vi "设备配置界面.vi"() -> ()   [LabVIEW 2016, in "环境动力监测库.lvlib"]
panel:
  in  "配置说明":bool
  in  "设置默认配置":bool
  in  "一键恢复默认设置":bool
  in  "add2":bool
  in  "串口连接":T1(ring)
  in  "设备列表":i32(listbox)=-1
  in  "add":bool
  in  "IO连接":T2(ring)
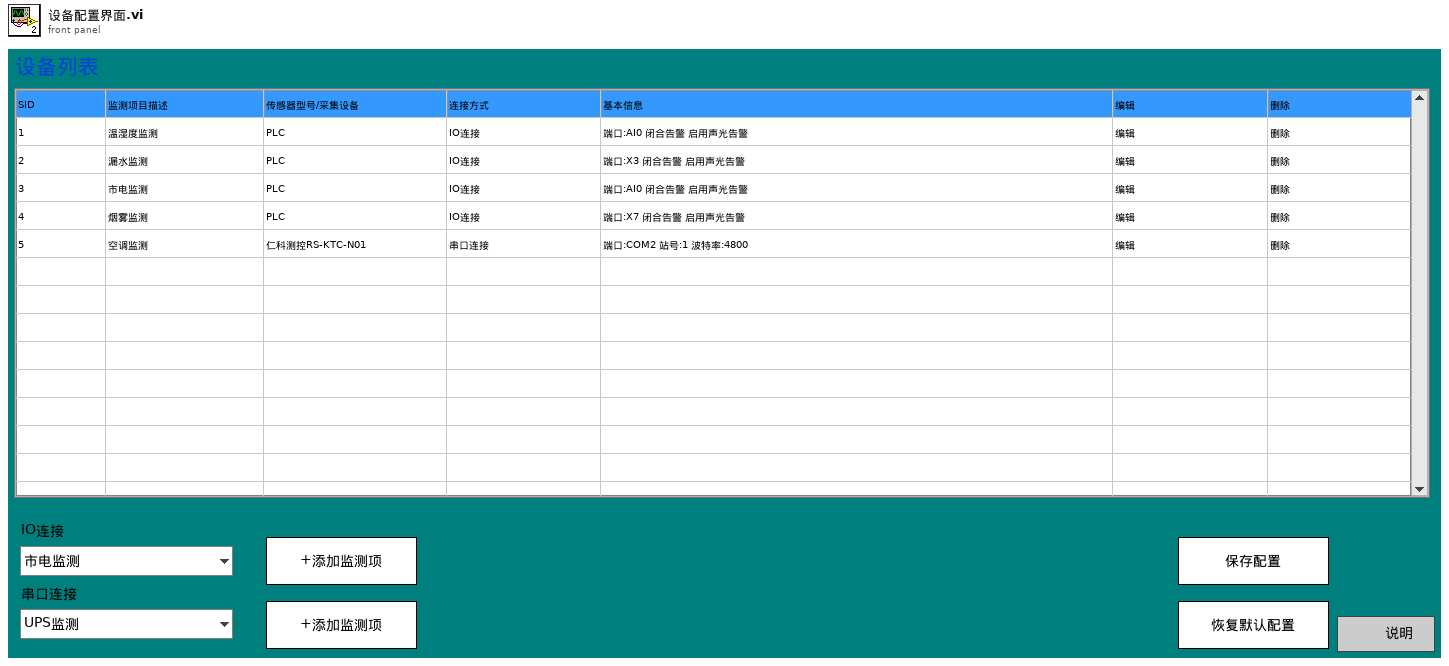
[diagram p1: front panel]
types:
  T1 = enum16{"UPS监测", "空调监测", "蓄电池监测", "GPS监测", "北斗监测", "智能门禁监测"}
  T2 = enum16{"市电监测", "用水量监测", "烟雾监测", "温湿度监测", "振动监测", "红外入侵监测", "漏水监测", "门禁开关监测", "视频监测", "冰箱监测", "排气扇监测"}
  T3 = cluster{"监测项描述:输出":string, "端口":enum16{"AI0", "AI1", "AI2", "AI3", "AI4", "DI0", "DI1", "DI2", "DI3", "DI4", "DO0", "DO1", "DO2", "DO3", "DO4", "X0", "X1", "X2", "X3", "X4", "X5", "X6", "X7", "X8", "X9", "X10", "X11", "X12", "X13", "X14", "X15", "X16", "X17", "X18", "X19", "X20", "X21", "X22", "X23"}, "告警方式":enum32{"禁用告警", "闭合告警", "断开告警"}, "传感器型号":enum16{"PLC", "ZLAN", "ART"}, "声光告警启用":bool}
  T4 = enum16{"AI0", "AI1", "AI2", "AI3", "AI4", "DI0", "DI1", "DI2", "DI3", "DI4", "DO0", "DO1", "DO2", "DO3", "DO4", "X0", "X1", "X2", "X3", "X4", "X5", "X6", "X7", "X8", "X9", "X10", "X11", "X12", "X13", "X14", "X15", "X16", "X17", "X18", "X19", "X20", "X21", "X22", "X23"}
  T5 = cluster{"监测项描述:输出":string, "连接方式":enum16{"串口", "TCP"}, "端口":string, "IP address:":string, "Port:":string, "站号":u64, "传感器型号":string, "波特率":u64, "data bits":u64, "停止位":u16, "奇偶校验":u16, "声光告警启用":bool}
  T6 = typedef "LVPoint32TypeDef.ctl" = cluster{"Horizontal":i32, "Vertical":i32}
  T7 = typedef "LVRowAndColumnTypeDef.ctl" = cluster{"Row":i32, "Column":i32}
  T8 = enum16{"Left Button", "Center Button", "Right Button", "Window Close"}
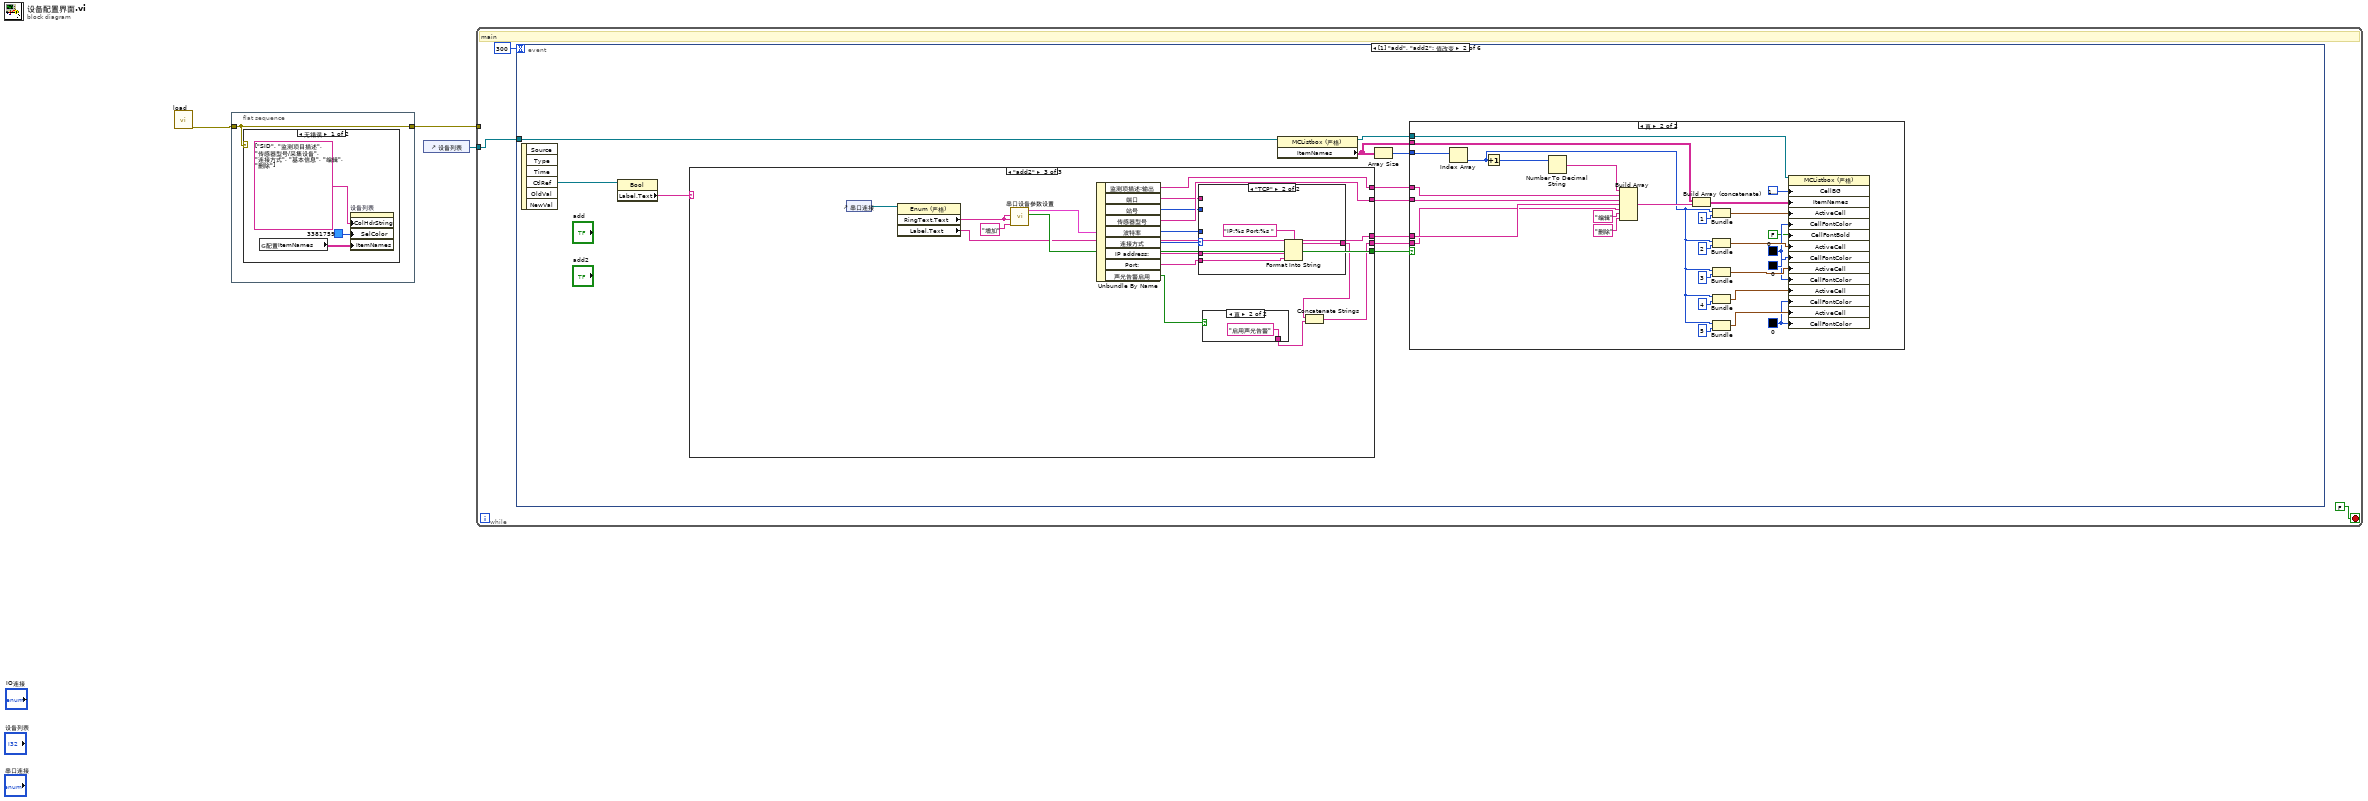
[diagram p0: block diagram]
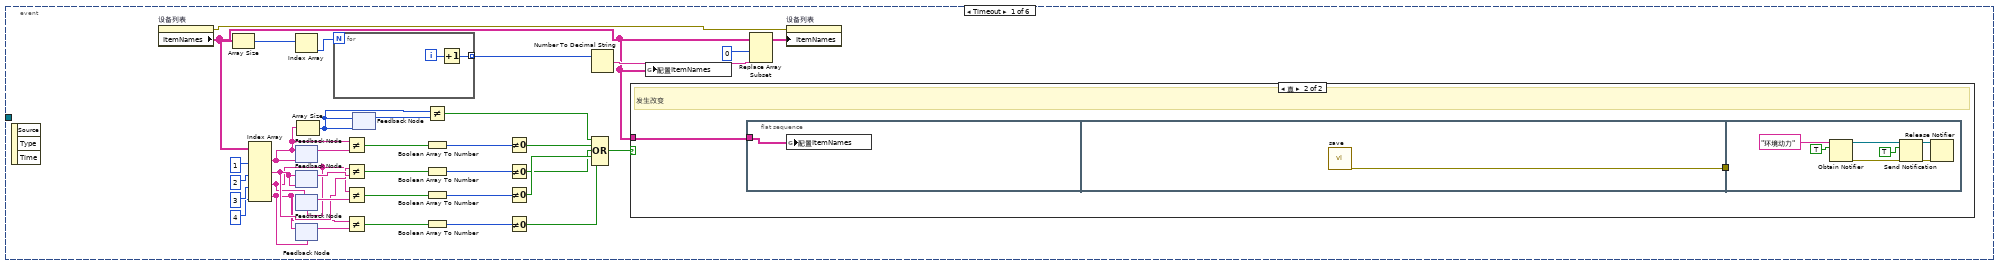
[diagram p3: hidden frame]
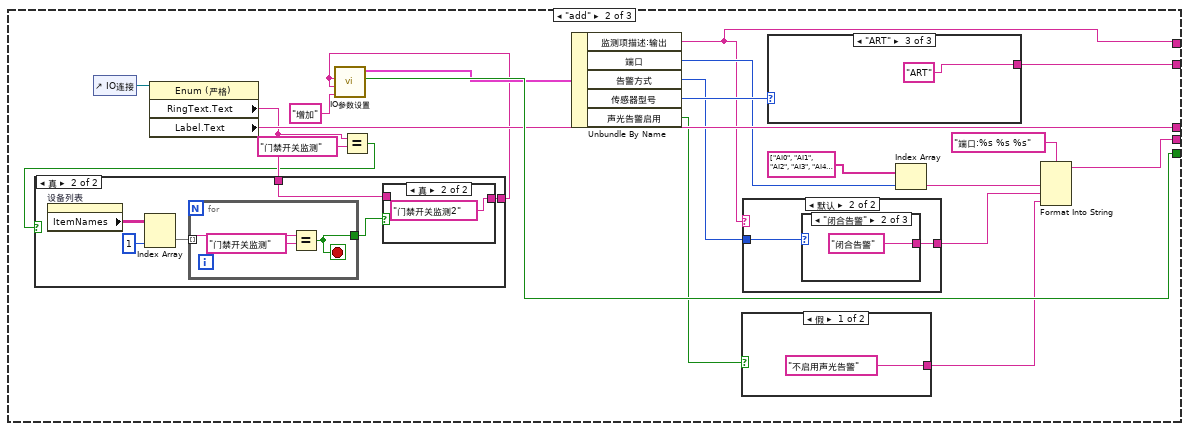
[diagram p6: hidden frame]
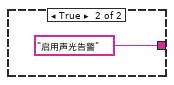
[diagram p7: hidden frame]
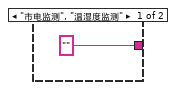
[diagram p10: hidden frame]
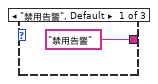
[diagram p11: hidden frame]
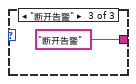
[diagram p12: hidden frame]
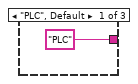
[diagram p13: hidden frame]
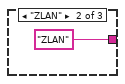
[diagram p14: hidden frame]
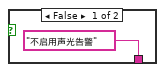
[diagram p15: hidden frame]
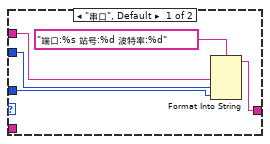
[diagram p16: hidden frame]
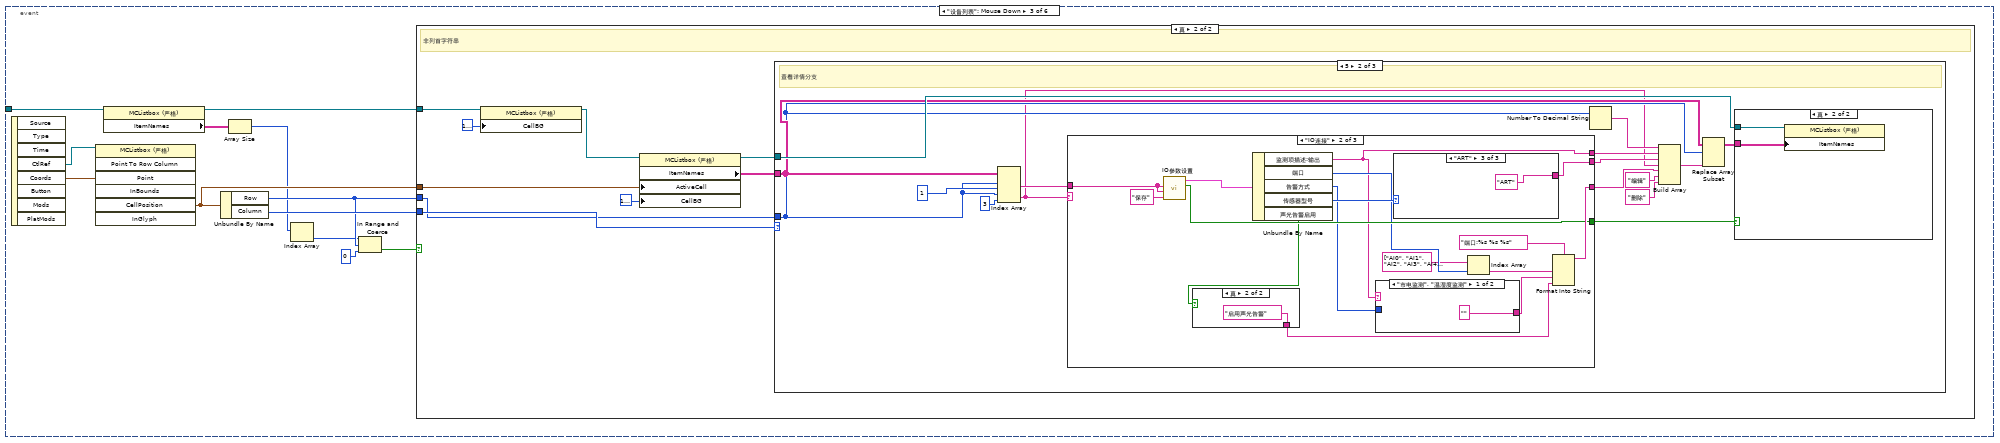
[diagram p18: hidden frame]
diagram:
  n1 = call "load.vi"() -> ("error out"=w1:errorcluster)  [unwired: 11 in]
  n2 = flat-sequence {
    tunnel: w1 -> [w4]
    tunnel: [w4] -> w2
    frame #0 {
      n3 = case shown="无错误" w4 {
        frame No Error {
          n4 = global read "断电保存全局变量.vi" "配置ItemNames"() -> (w5:string[][])
          n5 = property on="设备列表" class="MCListbox (严格)"("ColHdrString"=string[] ["SID", "监测项目描述", "传感器型号/采集设备", "连接方式", "基本信息", "编辑", "删除"] ("列首字符串[]"), "SelColor"=u32 3381759, "ItemNames"=w5) -> ()  [unwired: 2 in, 2 out]
        }
        frame Error {
        }
      }
    }
  }
  n6 = control-ref of="设备列表"() -> (w3:refnum<vi>)
  n7 = while {
    tunnel: w3 -> [w9]
    tunnel: w2 -> [_]
    stop <- FALSE stop-if-true
    # "main"
    n8 = event shown="[1] \"add\", \"add2\": 值改变" {
      selector: _ -> [_ _ _ _ _ _]
      dyn-events: _ -> [_ _ _ _ _ _]
      timeout: 300 -> [_ _ _ _ _ _]
      tunnel: w9 -> [_ w70 w178 _ _ _]
      event Timeout {
        n9 = event-data() -> ()  [unwired: 1 in, 3 out]
        n10 = property on="设备列表" class="MCListbox (严格)"() -> (error out=w45:errorcluster, "ItemNames"=w11:string[][])  [unwired: 2 in, 1 out]
        n11 = Array Size(array=w11) -> (size(s)=w46:i32[])
        n12 = Index Array(array=w11, index (col) #1=1 ("禁用的索引 (列)"), index (col) #2=2 ("索引 (列)"), index (col) #3=3 ("索引 (列)"), index (col) #4=4 ("索引 (列)")) -> (element #1=w16:string[], element #2=w23:string[], element #3=w22:string[], element #4=w21:string[])  [unwired: 4 in]
        n13 = Index Array(array=w46) -> (element=w40:i32)  [unwired: 1 in]
        n14 = feedback-in #1(w16) -> ()
        n15 = feedback #1(w16) -> (w35:string[])
        n16 = feedback #2(w23) -> (w30:string[])
        n17 = feedback-in #2(w23) -> ()
        n18 = feedback #3(w22) -> (w29:string[])
        n19 = feedback-in #3(w22) -> ()
        n20 = feedback #4(w21) -> (w24:string[])
        n21 = feedback-in #4(w21) -> ()
        n22 = Array Size(array=w16) -> (size(s)=w14:i32)
        n23 = for {
          N: w40 -> [_]
          tunnel: [w58] -> w44 mode=indexing
          i -> [w59]
          n24 = Increment(x=w59) -> (x+1=w58:i32)
        }
        n25 = Not Equal?(x=w16, y=w35) -> (x != y?=w15:bool[])
        n26 = Not Equal?(x=w23, y=w30) -> (x != y?=w31:bool[])
        n27 = Not Equal?(x=w22, y=w29) -> (x != y?=w28:bool[])
        n28 = Not Equal?(x=w21, y=w24) -> (x != y?=w25:bool[])
        n29 = feedback #5(w14) -> (w13:i32)
        n30 = feedback-in #5(w14) -> ()
        n31 = Not Equal?(x=w14, y=w13) -> (x != y?=w12:bool)
        n32 = Boolean Array To Number(Boolean array=w15) -> (number=w34:u32)
        n33 = Boolean Array To Number(Boolean array=w31) -> (number=w32:u32)
        n34 = Boolean Array To Number(Boolean array=w28) -> (number=w27:u32)
        n35 = Boolean Array To Number(Boolean array=w25) -> (number=w26:u32)
        n36 = Not Equal To 0?(x=w34) -> (x != 0?=w33:bool)
        n37 = Not Equal To 0?(x=w32) -> (x != 0?=w18:bool)
        n38 = Not Equal To 0?(x=w27) -> (x != 0?=w19:bool)
        n39 = Not Equal To 0?(x=w26) -> (x != 0?=w20:bool)
        n40 = Number To Decimal String(number=w44) -> (decimal integer string=w43:string[])  [unwired: 1 in]
        n41 = Compound Arithmetic op=OR ("复合运算")(w12, w33, w18, w19, w20) -> (w17:bool)
        n42 = case shown="真" w17 {
          tunnel: w11 -> [_ w48]
          frame False {
          }
          frame True {
            # "发生改变"
            n43 = flat-sequence {
              tunnel: w48 -> [w49]
              tunnel: [w50] -> w47
              tunnel: w47 -> [_]
              frame #0 {
                n44 = global write "断电保存全局变量.vi" "配置ItemNames"(w49) -> ()
              }
              frame #1 {
                n45 = call "save.vi"() -> ("error out"=w50:errorcluster)  [unwired: 11 in]
              }
              frame #2 {
                n46 = Obtain Notifier(name (unnamed)="环境动力" ("名称（未命名）"), notification data type=TRUE) -> (notifier out=w53:refnum<notifier>, error out=w54:errorcluster)  [unwired: 2 in, 1 out]
                n47 = Send Notification(notification=TRUE ("通知"), notifier=w53, error in (no error)=w54) -> (notifier out=w56:refnum<notifier>, error out=w57:errorcluster)
                n48 = Release Notifier(notifier=w56, error in (no error)=w57) -> ()  [unwired: 1 in, 3 out]
              }
            }
          }
        }
        n49 = global write "断电保存全局变量.vi" "配置ItemNames"(w11) -> ()
        n50 = Replace Array Subset(array=w11, new element=w43, index (col)=0 ("禁用的索引 (列)")) -> (w41:string[][])  [unwired: 1 in]
        n51 = property on="设备列表" class="MCListbox (严格)"(error in=w45, "ItemNames"=w41) -> ()  [unwired: 1 in, 2 out]
      }
      event "add", "add2": Value Change {
        n52 = event-data() -> ("CtlRef"=w65:refnum<vi>)  [unwired: 1 in, 5 out]
        n53 = property class="Bool"(reference=w65) -> ("Label.Text"=w64:string)  [unwired: 1 in, 2 out]
        n54 = case shown="\"add2\"" w64 {
          tunnel: [_ w91 w131] -> w67
          tunnel: [_ w88 w128] -> w63
          tunnel: [_ w78 w126] -> w62
          tunnel: [_ w83 w125] -> w61
          tunnel: [_ w85 w115] -> w60
          frame "假", Default {
          }
          frame "add" {
            n55 = control-ref of="IO连接"() -> (w89:refnum<vi>)
            n56 = property class="Enum (严格)"(reference=w89) -> ("RingText.Text"=w75:string, "Label.Text"=w88:string)  [unwired: 1 in, 2 out]
            n57 = Equal?(x=w75, y="门禁开关监测") -> (x = y?=w74:bool)
            n58 = case shown="真" w74 {
              tunnel: [w94 w97] -> w77
              tunnel: w75 -> [w94 w96]
              frame False {
              }
              frame True {
                n59 = property on="设备列表" class="MCListbox (严格)"() -> ("ItemNames"=w100:string[][])  [unwired: 2 in, 2 out]
                n60 = Index Array(array=w100, index (col)=1 ("禁用的索引 (列)")) -> (element=w98:string[])  [unwired: 1 in]
                n61 = for {
                  tunnel: w98 -> [w105] mode=indexing
                  tunnel: [w103] -> w95
                  stop <- w103 stop-if-true
                  n62 = Equal?(x=w105, y="门禁开关监测") -> (x = y?=w103:bool)
                }
                n63 = case shown="真" w95 {
                  tunnel: w96 -> [w101 _]
                  tunnel: [w101 "门禁开关监测2" ("y")] -> w97
                  frame False {
                  }
                  frame True {
                  }
                }
              }
            }
            n64 = call "IO参数设置.vi"("布尔文本.文本"="增加", "section (optional)"=w77, "监测项描述"=w77) -> ("增加？"=w91:bool, "簇1输出"=w87:T3)  [unwired: 7 in]
            n65 = Unbundle By Name(w87) -> ("监测项描述:输出"=w78:string, "端口"=w82:T4, "告警方式"=w80:enum32{"禁用告警", "闭合告警", "断开告警"}, "传感器型号"=w84:enum16{"PLC", "ZLAN", "ART"}, "声光告警启用"=w73:bool)
            n66 = case shown="假" w73 {
              tunnel: ["不启用声光告警" "启用声光告警"] -> w72
              frame False {
              }
              frame True {
              }
            }
            n67 = case shown="默认" w78 {
              tunnel: w80 -> [_ w108]
              tunnel: ["" w107] -> w79
              frame "市电监测", "温湿度监测" {
              }
              frame Default {
                n68 = case shown="\"闭合告警\"" w108 {
                  tunnel: ["禁用告警" "闭合告警" "断开告警"] -> w107
                  frame "禁用告警", Default {
                  }
                  frame "闭合告警" {
                  }
                  frame "断开告警" {
                  }
                }
              }
            }
            n69 = case shown="\"ART\"" w84 {
              tunnel: ["PLC" "ZLAN" "ART"] -> w83
              frame "PLC", Default {
              }
              frame "ZLAN" {
              }
              frame "ART" {
              }
            }
            n70 = Index Array(array=string[] ["AI0", "AI1", "AI2", "AI3", "AI4", "DI0", "DI1", "DI2", "DI3", "DI4", "DO0", "DO1", "DO2", "DO3", "DO4", "X0", "X1", "X2", "X3", "X4", "X5", "X6", "X7", "X8", "X9", "X10", "X11", "X12", "X13", "X14", "X15", "X16", "X17", "X18", "X19", "X20", "X21", "X22", "X23"] ("字符串[]"), index=w82) -> (element=w81:string)
            n71 = Format Into String(format string="端口:%s %s %s" ("格式字符串"), w81, w79, w72) -> (resulting string=w85:string)  [unwired: 2 in, 1 out]
          }
          frame "add2" {
            n72 = control-ref of="串口连接"() -> (w129:refnum<vi>)
            n73 = property class="Enum (严格)"(reference=w129) -> ("RingText.Text"=w130:string, "Label.Text"=w128:string)  [unwired: 1 in, 2 out]
            n74 = call "串口设备参数设置.vi"("布尔文本.文本"="增加" ("section (optional)"), "section (optional)"=w130, "监测项描述"=w130) -> ("布尔"=w131:bool, "输出簇"=w127:T5)  [unwired: 7 in]
            n75 = Unbundle By Name(w127) -> ("监测项描述:输出"=w126:string, "端口"=w123:string, "站号"=w122:u64, "传感器型号"=w125:string, "波特率"=w121:u64, "连接方式"=w124:enum16{"串口", "TCP"}, "IP address:"=w120:string, "Port:"=w119:string, "声光告警启用"=w118:bool)
            n76 = case shown="\"TCP\"" w124 {
              tunnel: [w138 w140] -> w116
              tunnel: w123 -> [w137 _]
              tunnel: w122 -> [w136 _]
              tunnel: w121 -> [w135 _]
              tunnel: w120 -> [_ w142]
              tunnel: w119 -> [_ w141]
              frame "串口", Default {
                n77 = Format Into String(format string="端口:%s 站号:%d 波特率:%d" ("格式字符串"), w137, w136, w135) -> (resulting string=w138:string)  [unwired: 2 in, 1 out]
              }
              frame "TCP" {
                n78 = Format Into String(format string="IP:%s Port:%s " ("格式字符串"), w142, w141) -> (resulting string=w140:string)  [unwired: 2 in, 1 out]
              }
            }
            n79 = case shown="真" w118 {
              tunnel: ["不启用声光告警" ("格式字符串") "启用声光告警" ("格式字符串")] -> w117
              frame False {
              }
              frame True {
              }
            }
            n80 = Concatenate Strings(w116, w117) -> (w115:string)
          }
        }
        n81 = property class="MCListbox (严格)"(reference=w70) -> (reference out=w68:refnum<vi>, "ItemNames"=w66:string[][])  [unwired: 1 in, 1 out]
        n82 = Array Size(array=w66) -> (size(s)=w69:i32[])
        n83 = case shown="真" w67 {
          tunnel: w66 -> [_ w171]
          tunnel: w69 -> [_ w170]
          tunnel: w68 -> [_ w168]
          tunnel: w63 -> [_ w150]
          tunnel: w62 -> [_ w147]
          tunnel: w61 -> [_ w146]
          tunnel: w60 -> [_ w145]
          frame False {
          }
          frame True {
            w151 = u32 0 ("颜色盒")
            w158 = u32 0 ("颜色盒")
            n84 = Index Array(array=w170) -> (element=w153:i32)  [unwired: 1 in]
            n85 = Increment(x=w153) -> (x+1=w169:i32)
            n86 = Number To Decimal String(number=w169) -> (decimal integer string=w148:string)  [unwired: 1 in]
            n87 = Build Array(w148, w147, w146, w150, w145, "编辑" ("元素"), "删除" ("元素")) -> (w172:string[])
            n88 = Build Array (concatenate)(w171, w172) -> (w149:string[][])
            n89 = Bundle(w153, "Column"=1) -> (w159:cluster{i32, "Column":i32})  [unwired: 1 in]
            n90 = Bundle(w153, "Column"=2) -> (w165:cluster{i32, "Column":i32})  [unwired: 1 in]
            n91 = Bundle(w153, "Column"=3) -> (w162:cluster{i32, "Column":i32})  [unwired: 1 in]
            n92 = Bundle(w153, "Column"=4) -> (w160:cluster{i32, "Column":i32})  [unwired: 1 in]
            n93 = Bundle(w153, "Column"=5) -> (w152:cluster{i32, "Column":i32})  [unwired: 1 in]
            n94 = property class="MCListbox (严格)"(reference=w168, "CellBG"=u32 16777216 ("颜色盒"), "ItemNames"=w149, "ActiveCell"=w159, "CellFontColor"=w158, "CellFontBold"=FALSE ("活动单元格:单元格字体:斜体"), "ActiveCell"=w165, "CellFontColor"=u32 0 ("颜色盒"), "ActiveCell"=w162, "CellFontColor"=w158, "ActiveCell"=w160, "CellFontColor"=w151, "ActiveCell"=w152, "CellFontColor"=w151) -> ()  [unwired: 1 in, 2 out]
          }
        }
      }
      event "设备列表": Mouse Down {
        n95 = event-data() -> ("CtlRef"=w184:refnum<vi>, "Coords"=w182:T6)  [unwired: 1 in, 6 out]
        n96 = invoke class="MCListbox (严格)" method="Point To Row Column"(reference=w184, "Point"=w182) -> ("CellPosition"=w181:T7)  [unwired: 5 in, 6 out]
        n97 = property class="MCListbox (严格)"(reference=w178) -> (reference out=w174:refnum<vi>, "ItemNames"=w177:string[][])  [unwired: 1 in, 1 out]
        n98 = Unbundle By Name(w181) -> ("Row"=w180:i32, "Column"=w183:i32)
        n99 = Array Size(array=w177) -> (size(s)=w176:i32[])
        n100 = Index Array(array=w176) -> (element=w175:i32)  [unwired: 1 in]
        n101 = In Range and Coerce(upper limit=w175, x=w180, lower limit=0 ("下限")) -> (In Range?=w173:bool)  [unwired: 1 out]
        n102 = case shown="真" w173 {
          tunnel: w183 -> [_ w192]
          tunnel: w180 -> [_ w191]
          tunnel: w181 -> [_ w189]
          tunnel: w174 -> [_ w186]
          frame False {
          }
          frame True {
            # "非列首字符串"
            n103 = property class="MCListbox (严格)"(reference=w186, "CellBG"=u32 16777216) -> (reference out=w187:refnum<vi>)  [unwired: 1 in, 1 out]
            n104 = property class="MCListbox (严格)"(reference=w187, "ActiveCell"=w189, "CellBG"=u32 16777216) -> (reference out=w190:refnum<vi>, "ItemNames"=w193:string[][])  [unwired: 1 in, 1 out]
            n105 = case shown="5" w192 {
              tunnel: w193 -> [_ w205 w273]
              tunnel: w191 -> [_ w200 w271]
              tunnel: w190 -> [_ w206 w272]
              frame 0, Default {
              }
              frame 5 {
                # "查看详情分支"
                n106 = Index Array(array=w205, index (row) #1=w200, index (col) #1=1 ("禁用的索引 (列)"), index (row) #2=w200, index (col) #2=3 ("禁用的索引 (列)")) -> (element #1=w208:string, element #2=w195:string)
                n107 = case shown="\"IO连接\"" w195 {
                  tunnel: w208 -> [_ w222 w249]
                  tunnel: [_ w216 w252] -> w198
                  tunnel: [_ w224 w240] -> w196
                  tunnel: [_ w220 w251] -> w197
                  tunnel: [_ w223 w250] -> w194
                  frame "假", Default {
                  }
                  frame "IO连接" {
                    n108 = call "IO参数设置.vi"("布尔文本.文本"="保存", "section (optional)"=w222, "监测项描述"=w222) -> ("增加？"=w223:bool, "簇1输出"=w225:T3)  [unwired: 7 in]
                    n109 = Unbundle By Name(w225) -> ("监测项描述:输出"=w216:string, "端口"=w219:T4, "告警方式"=w217:enum32{"禁用告警", "闭合告警", "断开告警"}, "传感器型号"=w221:enum16{"PLC", "ZLAN", "ART"}, "声光告警启用"=w213:bool)
                    n110 = case shown="真" w213 {
                      tunnel: ["不启用声光告警" ("格式字符串") "启用声光告警" ("格式字符串")] -> w212
                      frame False {
                      }
                      frame True {
                      }
                    }
                    n111 = case shown="\"市电监测\", \"温湿度监测\"" w216 {
                      tunnel: w217 -> [_ w232]
                      tunnel: ["" w231] -> w215
                      frame "市电监测", "温湿度监测" {
                      }
                      frame Default {
                        n112 = case shown="\"禁用告警\", 默认" w232 {
                          tunnel: ["禁用告警" "闭合告警" "断开告警"] -> w231
                          frame "禁用告警", Default {
                          }
                          frame "闭合告警" {
                          }
                          frame "断开告警" {
                          }
                        }
                      }
                    }
                    n113 = case shown="\"ART\"" w221 {
                      tunnel: ["PLC" "ZLAN" "ART"] -> w220
                      frame "PLC", Default {
                      }
                      frame "ZLAN" {
                      }
                      frame "ART" {
                      }
                    }
                    n114 = Index Array(array=string[] ["AI0", "AI1", "AI2", "AI3", "AI4", "DI0", "DI1", "DI2", "DI3", "DI4", "DO0", "DO1", "DO2", "DO3", "DO4", "X0", "X1", "X2", "X3", "X4", "X5", "X6", "X7", "X8", "X9", "X10", "X11", "X12", "X13", "X14", "X15", "X16", "X17", "X18", "X19", "X20", "X21", "X22", "X23"] ("字符串[]"), index=w219) -> (element=w218:string)
                    n115 = Format Into String(format string="端口:%s %s %s" ("格式字符串"), w218, w215, w212) -> (resulting string=w224:string)  [unwired: 2 in, 1 out]
                  }
                  frame "串口连接" {
                    n116 = call "串口设备参数设置.vi"("布尔文本.文本"="保存", "section (optional)"=w249, "监测项描述"=w249) -> ("布尔"=w250:bool, "输出簇"=w253:T5)  [unwired: 7 in]
                    n117 = Unbundle By Name(w253) -> ("监测项描述:输出"=w252:string, "端口"=w245:string, "站号"=w244:u64, "传感器型号"=w251:string, "波特率"=w243:u64, "连接方式"=w246:enum16{"串口", "TCP"}, "IP address:"=w248:string, "Port:"=w247:string, "声光告警启用"=w242:bool)
                    n118 = case shown="真" w242 {
                      tunnel: ["不启用声光告警" ("格式字符串") "启用声光告警" ("格式字符串")] -> w239
                      frame False {
                      }
                      frame True {
                      }
                    }
                    n119 = case shown="\"TCP\"" w246 {
                      tunnel: [w260 w262] -> w241
                      tunnel: w245 -> [w259 _]
                      tunnel: w244 -> [w258 _]
                      tunnel: w243 -> [w257 _]
                      tunnel: w248 -> [_ w264]
                      tunnel: w247 -> [_ w263]
                      frame "串口", Default {
                        n120 = Format Into String(format string="端口:%s 站号:%d 波特率:%d" ("格式字符串"), w259, w258, w257) -> (resulting string=w260:string)  [unwired: 2 in, 1 out]
                      }
                      frame "TCP" {
                        n121 = Format Into String(format string="IP:%s Port:%s " ("格式字符串"), w264, w263) -> (resulting string=w262:string)  [unwired: 2 in, 1 out]
                      }
                    }
                    n122 = Concatenate Strings(w241, w239) -> (w240:string)
                  }
                }
                n123 = Number To Decimal String(number=w200) -> (decimal integer string=w199:string)  [unwired: 1 in]
                n124 = Build Array(w199, w198, w197, w195, w196, "编辑" ("元素"), "删除" ("元素")) -> (w201:string[])
                n125 = Replace Array Subset(array=w205, new element=w201, index (row)=w200) -> (w204:string[][])  [unwired: 1 in]
                n126 = case shown="真" w194 {
                  tunnel: w206 -> [_ w211]
                  tunnel: w204 -> [_ w210]
                  frame False {
                  }
                  frame True {
                    n127 = property class="MCListbox (严格)"(reference=w211, "ItemNames"=w210) -> ()  [unwired: 1 in, 2 out]
                  }
                }
              }
              frame 6 {
                # "删除"
                n128 = Index Array(array=w273, index (row)=w271, index (col)=1 ("禁用的索引 (列)")) -> (element=w267:string)
                n129 = Format Into String(format string="是否删除%s？" ("消息"), w267) -> (resulting string=w269:string)  [unwired: 2 in, 1 out]
                n130 = Two Button Dialog(message=w269) -> (T button?=w266:bool)  [unwired: 2 in]
                n131 = case shown="真" w266 {
                  tunnel: w272 -> [_ w278]
                  tunnel: w273 -> [_ w277]
                  tunnel: w271 -> [_ w276]
                  frame False {
                  }
                  frame True {
                    # "触发删除事件"
                    n132 = Delete From Array(array=w277, length=1 ("长度"), index (row)=w276) -> (array with subset deleted=w274:string[][])  [unwired: 1 in, 1 out]
                    n133 = property class="MCListbox (严格)"(reference=w278, "ItemNames"=w274) -> ()  [unwired: 1 in, 2 out]
                  }
                }
              }
            }
          }
        }
      }
      event "一键恢复默认设置": Value Change {
        n134 = event-data() -> ()  [unwired: 1 in, 6 out]
        n135 = call <vilib>:"Three Button Dialog.vi"("Center Button Text (\"No\")"="配置文件" ("Center Button Text (\"No\")"), "Left Button Text (\"Yes\")"="本机" ("Left Button Text (\"Yes\")"), "message"="请选择是否恢复默认？") -> ("Which Button?"=w280:T8)  [unwired: 8 in]
        n136 = case shown="\"Left Button\", 默认" w280 {
          frame "Left Button", Default {
            n137 = call "开机添加默认配置文件.vi"("恢复默认方式"=enum16{"无配置开机恢复", "手动恢复"}."手动恢复") -> ("error out"=w283:errorcluster)  [unwired: 10 in]
            n138 = case shown="无错误" w283 {
              frame No Error {
                n139 = One Button Dialog(message="配置成功！" ("消息")) -> (true=w285:bool)  [unwired: 1 in]
                n140 = case shown="真" w285 {
                  frame False {
                  }
                  frame True {
                    n141 = call "load.vi"() -> ("error out"=w287:errorcluster)  [unwired: 11 in]
                    n142 = flat-sequence {
                      tunnel: w287 -> [w288]
                      tunnel: [w288] -> _
                      frame #0 {
                        n143 = case shown="无错误" w288 {
                          frame No Error {
                            n144 = global read "断电保存全局变量.vi" "配置ItemNames"() -> (w290:string[][])
                            n145 = control-ref of="设备列表"() -> (w289:refnum<vi>)
                            n146 = property on="属性节点" class="MCListbox (严格)"(reference=w289, "ColHdrString"=string[] ["SID", "监测项目描述", "传感器型号/采集设备", "连接方式", "基本信息", "编辑", "删除"] ("列首字符串[]"), "SelColor"=u32 3381759, "ItemNames"=w290) -> ()  [unwired: 1 in, 2 out]
                          }
                          frame Error {
                          }
                        }
                      }
                    }
                  }
                }
              }
              frame Error {
                n147 = One Button Dialog(message="配置失败！" ("消息")) -> ()  [unwired: 1 in, 1 out]
              }
            }
          }
          frame "Center Button" {
            n148 = vi-ref "环境动力监测库.lvlib:断电保存全局变量.vi"() -> (w298:refnum<vi>)
            n149 = call "load config.vi"("TABLE"="power_environment_monitoring_default", "VI引用句柄"=w298) -> ("error out"=w295:errorcluster)  [unwired: 9 in]
            n150 = vi-ref "环境动力监测库.lvlib:断电保存全局变量.vi"() -> (w299:refnum<vi>)
            n151 = call "save config.vi"("error in (no error)"=w295, "TABLE"="power_environment_monitoring", "VI引用句柄"=w299) -> ("error out"=w294:errorcluster)  [unwired: 8 in]
            n152 = case shown="无错误" w294 {
              frame No Error {
                n153 = One Button Dialog(message="配置成功！" ("消息")) -> (true=w300:bool)  [unwired: 1 in]
                n154 = case shown="真" w300 {
                  frame False {
                  }
                  frame True {
                    n155 = call "load.vi"() -> ("error out"=w302:errorcluster)  [unwired: 11 in]
                    n156 = flat-sequence {
                      tunnel: w302 -> [w303]
                      tunnel: [w303] -> _
                      frame #0 {
                        n157 = case shown="无错误" w303 {
                          frame No Error {
                            n158 = global read "断电保存全局变量.vi" "配置ItemNames"() -> (w305:string[][])
                            n159 = control-ref of="设备列表"() -> (w304:refnum<vi>)
                            n160 = property on="属性节点" class="MCListbox (严格)"(reference=w304, "ColHdrString"=string[] ["SID", "监测项目描述", "传感器型号/采集设备", "连接方式", "基本信息", "编辑", "删除"] ("列首字符串[]"), "SelColor"=u32 3381759, "ItemNames"=w305) -> ()  [unwired: 1 in, 2 out]
                          }
                          frame Error {
                          }
                        }
                      }
                    }
                  }
                }
              }
              frame Error {
              }
            }
          }
          frame "Right Button" {
          }
          frame "Window Close" {
          }
        }
      }
      event "设置默认配置": Value Change {
        n161 = event-data() -> ()  [unwired: 1 in, 6 out]
        n162 = Two Button Dialog(message="确认将当前配置设置为默认配置？" ("消息")) -> (T button?=w308:bool)  [unwired: 2 in]
        n163 = case shown="真" w308 {
          frame False {
          }
          frame True {
            n164 = vi-ref "环境动力监测库.lvlib:断电保存全局变量.vi"() -> (w312:refnum<vi>)
            n165 = call "save config.vi"("TABLE"="power_environment_monitoring_default", "VI引用句柄"=w312) -> ("error out"=w310:errorcluster)  [unwired: 9 in]
            n166 = case shown="无错误" w310 {
              frame No Error {
                n167 = One Button Dialog(message="配置成功！" ("消息")) -> ()  [unwired: 1 in, 1 out]
              }
              frame Error {
                n168 = One Button Dialog(message="配置失败！" ("消息")) -> ()  [unwired: 1 in, 1 out]
              }
            }
          }
        }
      }
      event "配置说明": Value Change {
        n169 = event-data() -> ()  [unwired: 1 in, 6 out]
        n170 = vi-ref "环境动力监测库.lvlib:配置说明.vi"() -> (w315:refnum<vi>)
        n171 = property class="VI"(reference=w315) -> ("Name"=w316:string)  [unwired: 1 in, 2 out]
        n172 = Open VI Reference(type specifier VI Refnum (for type only)=refnum<vi> refnum, vi path=w316, options=128 ("选项")) -> (vi reference=w318:refnum<vi>, error out=w320:errorcluster)  [unwired: 3 in]
        n173 = call-by-ref "开始异步调用"(reference=w318, error in=w320) -> (reference out=w322:refnum<vi>, error out=w321:errorcluster)  [unwired: 11 in, 1 out]
        n174 = Close Reference(reference=w322, error in (no error)=w321) -> ()  [unwired: 1 out]
      }
    }
  }
